vi "Initialize.vi"(8 "error in (no error)":errorcluster, 11 "FLOM Settings in":T1={"VISA resource name"="", "Simulated?"=FALSE, "Pump Number"=1.0} {"Pump Number" min=1.0 max=20.0 step=1.0}) -> (0 "error out":errorcluster, 1 "Initialized":bool, 2 "No Pump Connected":bool, 3 "FLOM Settings out":T1={"VISA resource name"="", "Simulated?"=FALSE, "Pump Number"=1.0} {"Pump Number" min=1.0 max=20.0 step=1.0})   [LabVIEW 2018, in "FLOM Pump.lvlib"]
uses:
  FLOM Pump.lvlib
  Settings Cluster.ctl
  <vilib>/Instr/_visa.llb/VISA Configure Serial Port (Instr).vi
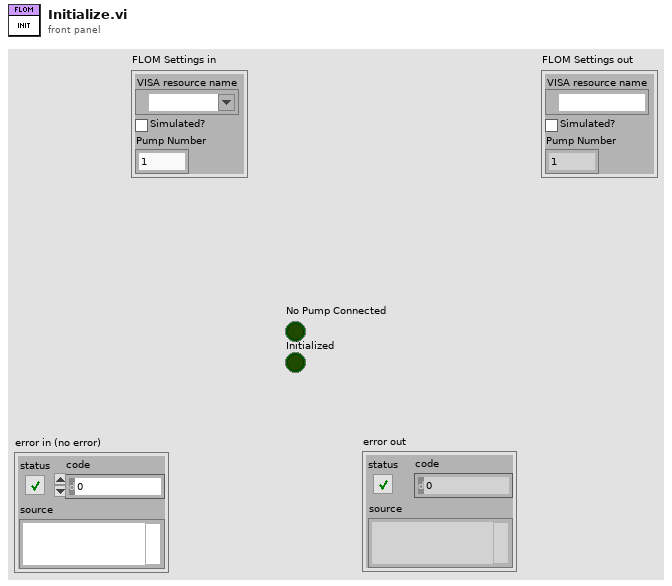
[diagram p1: front panel]
types:
  T1 = typedef "FLOM Pump.lvlib/Settings Cluster.ctl" = cluster{"VISA resource name":refnum<visa-resource-name>, "Simulated?":bool, "Pump Number":dbl}
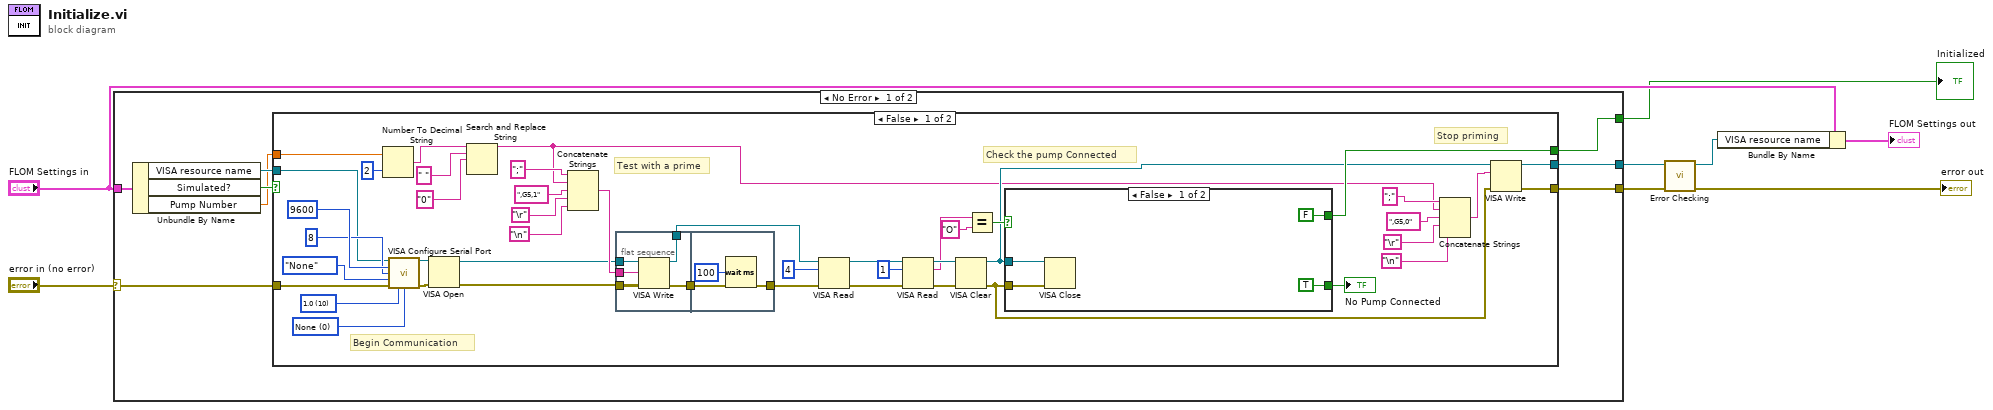
[diagram p0: block diagram]
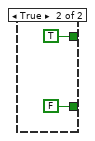
[diagram p2: hidden frame]
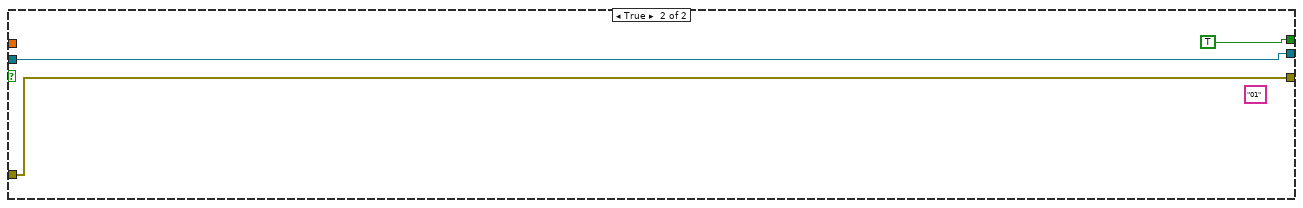
[diagram p3: hidden frame]
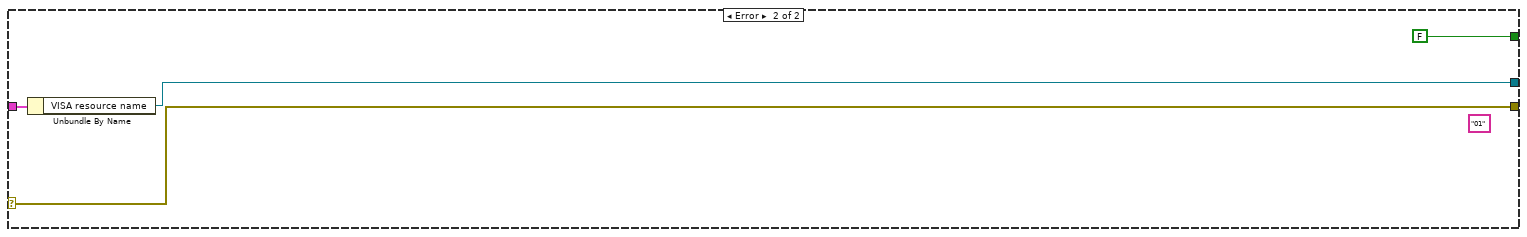
[diagram p4: hidden frame]
diagram:
  n1 = case shown="No Error" "error in (no error)" {
    selector: "error in (no error)" -> [w16 w81]
    tunnel: "FLOM Settings in" -> [w11 w80]
    tunnel: [w12 w81] -> w6
    tunnel: [w10 w79] -> w1
    tunnel: [w9 FALSE] -> w3
    frame No Error {
      n2 = Unbundle By Name(w11) -> ("VISA resource name"=w14:refnum<visa-resource-name>, "Simulated?"=w15:bool, "Pump Number"=w13:dbl)
      n3 = case shown="False" w15 {
        tunnel: w16 -> [w55 w77]
        tunnel: w14 -> [w53 w76]
        tunnel: w13 -> [w50 _]
        tunnel: [w19 w77] -> w12
        tunnel: [w17 w76] -> w10
        tunnel: [w44 TRUE] -> w9
        frame False {
          w57 = u16 0 items=["None", "XON/XOFF", "RTS/CTS", "XON/XOFF & RTS/CTS", "DTR/DSR", "XON/XOFF & DTR/DSR"] ("flow control (0:none)")
          w58 = u16 10 items=["1.0"=10, "1.5"=15, "2.0"=20] ("stop bits (10: 1 bit)")
          # "Stop priming"
          # "Test with a prime"
          # "Check the pump Connected"
          # "Begin Communication"
          n4 = Number To Decimal String(number=w50, width (-)=i16 2) -> (decimal integer string=w32:string)
          n5 = call-poly "VISA Configure Serial Port"("VISA resource name"=w53, "baud rate (9600)"=u32 9600, "data bits (8)"=u16 8, "parity (0:none)"=enum16{"None", "Odd", "Even", "Mark", "Space"}."None", "error in (no error)"=w55, "stop bits (10: 1 bit)"=w58, "flow control (0:none)"=w57) -> ("VISA resource name out"=w54:refnum<visa-resource-name>, "error out"=w56:errorcluster)  [unwired: 7 in]
          n6 = VISA Open(error in (no error)=w56, VISA resource name=w54) -> (VISA resource name=w28:refnum<visa-resource-name>, error out=w43:errorcluster)  [unwired: 3 in]
          n7 = Search and Replace String(input string=w32, search string=" ", replace string="0" ("replace string (\"\")")) -> (result string=w18:string)  [unwired: 5 in, 3 out]
          n8 = Concatenate Strings(";" ("string"), w18, ",G5,1" ("string"), "\r", "\n") -> (w51:string)
          n9 = flat-sequence {
            tunnel: w51 -> [w66]
            tunnel: w43 -> [w64]
            tunnel: [w65] -> w29
            tunnel: w28 -> [w63]
            tunnel: [w62] -> w27
            tunnel: [w68] -> w48
            tunnel: w29 -> [w68]
            frame #0 {
              n10 = VISA Write(VISA resource name=w63, write buffer=w66, error in (no error)=w64) -> (VISA resource name out=w62:refnum<visa-resource-name>, error out=w65:errorcluster)  [unwired: 1 out]
            }
            frame #1 {
              n11 = Wait (ms)(milliseconds to wait=u32 100) -> ()  [unwired: 1 out]
            }
          }
          n12 = VISA Read(VISA resource name=w27, byte count=u32 4, error in (no error)=w48) -> (VISA resource name out=w39:refnum<visa-resource-name>, error out=w38:errorcluster)  [unwired: 2 out]
          n13 = VISA Read(VISA resource name=w39, byte count=u32 1, error in (no error)=w38) -> (VISA resource name out=w37:refnum<visa-resource-name>, read buffer=w35:string, error out=w36:errorcluster)  [unwired: 1 out]
          n14 = VISA Clear(VISA resource name=w37, error in (no error)=w36) -> (VISA resource name out=w21:refnum<visa-resource-name>, error out=w20:errorcluster)
          n15 = Equal?(x=w35, y="O") -> (x = y?=w47:bool)
          n16 = case shown="False" w47 {
            tunnel: w21 -> [w72 _]
            tunnel: w20 -> [w71 _]
            tunnel: [TRUE FALSE] -> w45
            tunnel: [FALSE TRUE] -> w44
            frame False {
              n17 = VISA Close(VISA resource name=w72, error in (no error)=w71) -> ()  [unwired: 1 out]
            }
            frame True {
            }
          }
          "No Pump Connected" <- w45
          n18 = Concatenate Strings(";" ("string"), w18, ",G5,0" ("string"), "\r", "\n") -> (w26:string)
          n19 = VISA Write(VISA resource name=w21, write buffer=w26, error in (no error)=w20) -> (VISA resource name out=w17:refnum<visa-resource-name>, error out=w19:errorcluster)  [unwired: 1 out]
        }
        frame True {
          (unwired) "01" ("result string")
        }
      }
    }
    frame Error {
      (unwired) "01" ("result string")
      n20 = Unbundle By Name(w80) -> ("VISA resource name"=w79:refnum<visa-resource-name>)
    }
  }
  "Initialized" <- w3
  n21 = call "Error Checking.vi"("error in (no error)"=w6, "VISA resource name"=w1) -> ("error out"=→"error out":errorcluster, "VISA resource name"=w7:refnum<visa-resource-name>)  [unwired: 7 in, 1 out]
  n22 = Bundle By Name(cluster="FLOM Settings in", "VISA resource name"=w7) -> (→"FLOM Settings out":T1)
